vi "robot get param.vi"(0 "robot_id":i32, 11 "error in (no error)":errorcluster caption="错误输入（无错误）") -> (4 "robot_id out":i32, 6 "function return":i32, 8 "输出参数簇":T1, 15 "error out":errorcluster caption="错误输出")   [LabVIEW 2020, in "small_scara_interface.lvlib"]
doc: "extern \"C\" __declspec(dllexport) int robot_get_param(int robot_id, float* x, float* y, float* z, float* angle1, float* angle2, float* rotation, bool* communicate_success, bool* move_flag);"
uses:
  small_scara_interface.lvlib
  small_scara_interface.dll
panel:
  out "initial_finish out":bool
  in  "initial_finish":bool
  in  "move_flag":bool
  out "move_flag out":bool
  in  "communicate_success":bool
  out "communicate_success out":bool
  in  "rotation":sgl
  out "rotation out":sgl
  in  "angle2":sgl
  out "angle2 out":sgl
  in  "angle1":sgl
  out "angle1 out":sgl
  in  "z":sgl
  out "z out":sgl
  in  "y":sgl
  out "y out":sgl
  in  "x":sgl
  out "x out":sgl
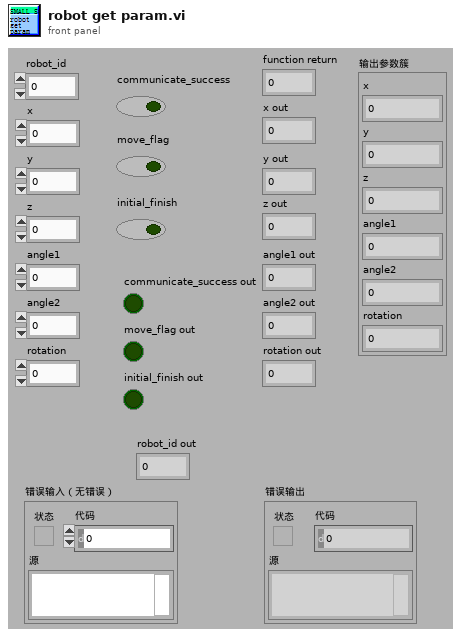
[diagram p1: front panel]
types:
  T1 = cluster{"x":sgl, "y":sgl, "z":sgl, "angle1":sgl, "angle2":sgl, "rotation":sgl}
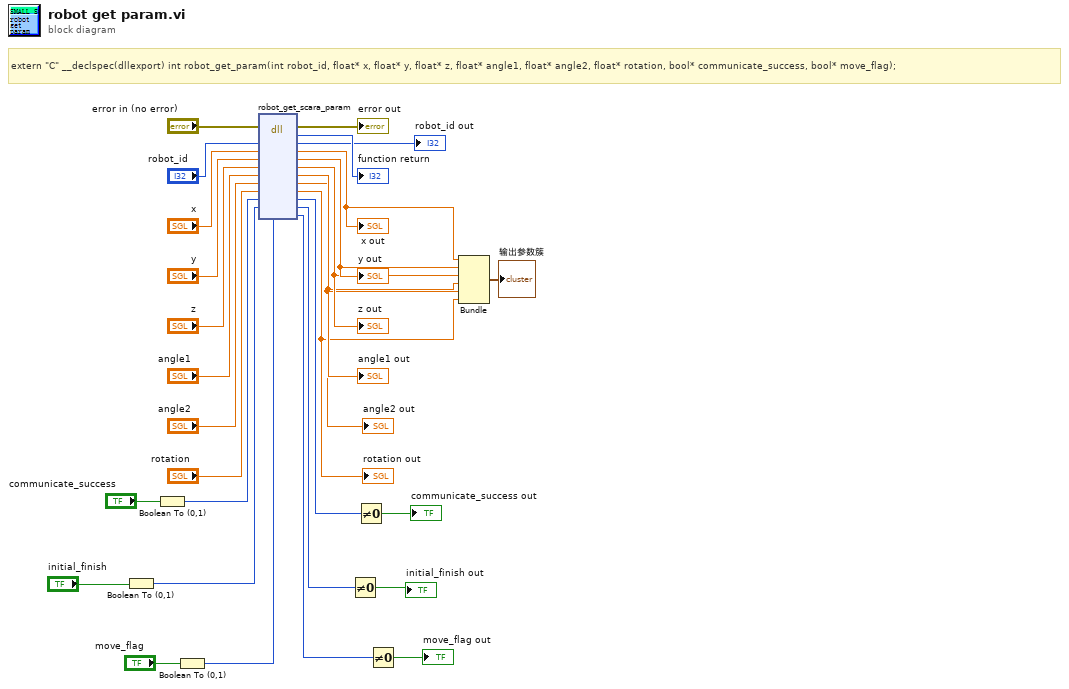
[diagram p0: block diagram]
diagram:
  # "extern \"C\" __declspec(dllexport) int robot_get_param(int robot_id, float* x, float* y, float* z, float* angle1, float* angle2, float* rotation, bool* communicate_success, bool* move_flag);"
  n1 = Boolean To (0,1)(Boolean="initial_finish") -> (0, 1=w3:i16)
  n2 = Boolean To (0,1)(Boolean="communicate_success") -> (0, 1=w21:i16)
  n3 = Boolean To (0,1)(Boolean="move_flag") -> (0, 1=w17:i16)
  n4 = dll-call lib="PTH2¦abs CUsers\tMogroup-3Desktopé›·èµ›Screening systemlabview multichannel v314subvirobotsubviRobot-HLsmall_scara_interfacesmall_scara_interface.*" fn="robot_get_scara_param"(error in="error in (no error)", "robot_id"="robot_id", "x"="x", "y"="y", "z"="z", "angle1"="angle1", "angle2"="angle2", "rotation"="rotation", "communicate_success"=w21, "initial_finsh"=w3, "move_flag"=w17) -> (error out=→"error out":errorcluster, "返回类型"=→"function return":i32, "robot_id"=→"robot_id out":i32, "x"=w12:sgl, "y"=w11:sgl, "z"=w10:sgl, "angle1"=w9:sgl, "angle2"=w8:sgl, "rotation"=w7:sgl, "communicate_success"=w19:u8, "initial_finsh"=w1:u8, "move_flag"=w15:u8)  [unwired: 2 in, 1 out]
  "x out" <- w12
  "y out" <- w11
  "z out" <- w10
  "angle1 out" <- w9
  "angle2 out" <- w8
  "rotation out" <- w7
  n5 = Not Equal To 0?(x=w1) -> (x != 0?=→"initial_finish out":bool)
  n6 = Not Equal To 0?(x=w19) -> (x != 0?=→"communicate_success out":bool)
  n7 = Not Equal To 0?(x=w15) -> (x != 0?=→"move_flag out":bool)
  n8 = Bundle("x"=w12, "y"=w11, "z"=w10, "angle1"=w9, "angle2"=w8, "rotation"=w7) -> (→"输出参数簇":T1)  [unwired: 1 in]
